vi "append_data.vi"(8 "error in (no error)":errorcluster, 10 "Array of ROI sums":dbl[][](array[numeric]), 11 "Camera in":refnum<class "Camera.lvclass">) -> (0 "error out":errorcluster, 3 "Camera out":refnum<class "Camera.lvclass">)   [LabVIEW 2013, in "Camera.lvclass"]
uses:
  Camera.lvclass
  Camera.lvclass/Camera.ctl
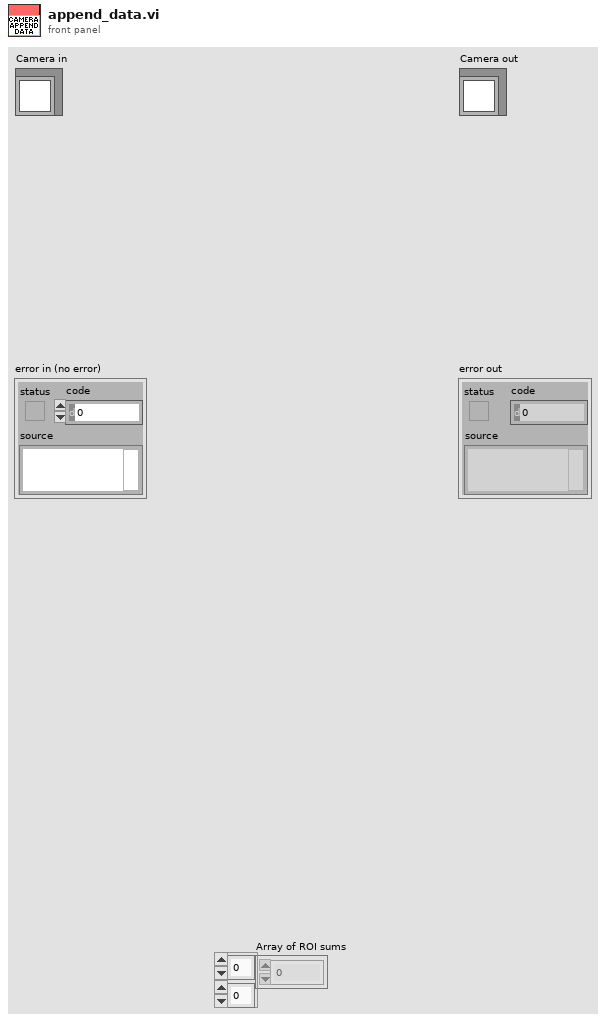
[diagram p1: front panel]
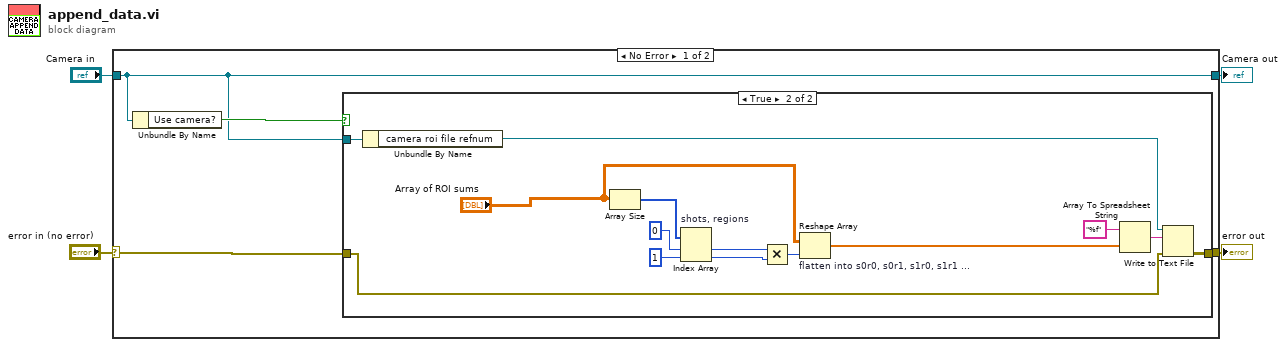
[diagram p0: block diagram]
diagram:
  n1 = case shown="No Error" "error in (no error)" {
    selector: "error in (no error)" -> [w8 w25]
    tunnel: [w7 w25] -> w3
    tunnel: [w5 w24] -> w1
    tunnel: "Camera in" -> [w5 w24]
    frame No Error {
      n2 = Unbundle By Name(w5) -> ("Use camera?"=w6:bool)
      n3 = case shown="True" w6 {
        tunnel: w8 -> [w9 w18]
        tunnel: [w9 w21] -> w7
        tunnel: w5 -> [_ w20]
        frame False {
        }
        frame True {
          n4 = Unbundle By Name(w20) -> ("camera roi file refnum"=w19:refnum<file>)
          n5 = Array Size(array="Array of ROI sums") -> (size(s)=w16:i32[])
          n6 = Index Array "shots, regions"(array=w16, index #1=0 ("index"), index #2=1 ("index")) -> (element #1=w13:i32, element #2=w12:i32)
          n7 = Multiply(x=w13, y=w12) -> (x*y=w11:i32)
          n8 = Reshape Array "flatten into s0r0, s0r1, s1r0, s1r1 ..."("Array of ROI sums", w11) -> (w10:dbl[])
          n9 = Array To Spreadsheet String(array=w10, 3:"%f" ("format string")) -> (spreadsheet string=w17:string)  [unwired: 1 in]
          n10 = Write to Text File(file (use dialog)=w19, text=w17, error in=w18) -> (error out=w21:errorcluster)  [unwired: 1 in, 2 out]
        }
      }
    }
    frame Error {
    }
  }
  "error out" <- w3
  "Camera out" <- w1
